vi "Poll Sensor Group 2.vi"(8 "error in":errorcluster, 11 "UART port in":T3) -> (0 "error out":errorcluster, 1 "Timed Out?":bool, 2 "Sensor Group 2":T1={"Infrared"=255, "Buttons"={"Advance"=FALSE, "Play"=FALSE}, "Distance (mm)"=0, "Angle (deg)"=0} {"Infrared" format="%02x"}, 3 "UART port out":T3)   [LabVIEW 2013]
doc: "Poll the iRobot for Sensor Group 2; blocks until response is received, or the operation has timed out.\n\nThis VI both writes to AND reads from the serial port.\n<b>NOTE</b>: This should not be used in a loop if other serial reading or writing VIs are called in parallel loops."
uses:
  Advanced/UART/iRobot UART Port Type.ctl
  Sensor Group 2.ctl
  Buttons.ctl
  Sensor ID.ctl
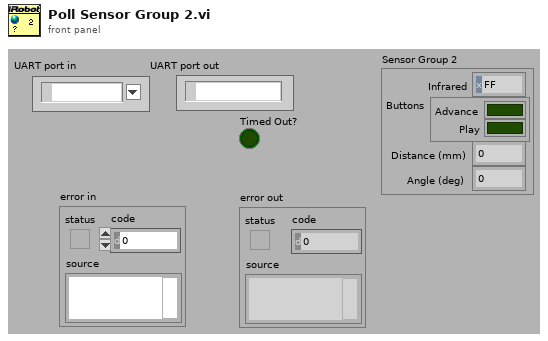
[diagram p1: front panel]
types:
  T1 = typedef "Sensor Group 2.ctl" = cluster{"Infrared":u8, "Buttons":T2, "Distance (mm)":i32, "Angle (deg)":i32}
  T2 = typedef "Buttons.ctl" = cluster{"Advance":bool, "Play":bool}
  T3 = typedef "iRobot UART Port Type.ctl" = refnum<visa-resource-name>
  T4 = typedef "Sensor ID.ctl" = enum8{"Sensor Group 0", "Sensor Group 1", "Sensor Group 2", "Sensor Group 3", "Sensor Group 4", "Sensor Group 5", "Sensor Group 6", "Bump + Wheel Drop", "Wall", "Cliff Left", "Cliff Front Left", "Cliff Front Right", "Cliff Right", "Virtual Wall", "Low Side Driver + Wheel Overcurrent", "Unused 0", "Unused 1", "Infrared", "Buttons", "Distance", "Angle", "Charging State", "Voltage", "Current", "Battery Temperature", "Battery Charge", "Battery Capacity", "Wall Signal", "Cliff Left Signal", "Cliff Front Left Signal", "Cliff Front Right Signal", "Cliff Right Signal", "Cargo Bay Digital Inputs", "Cargo Bay Analog Signal", "Charging Sources Available", "OI Mode", "Song Number", "Song Playing", "Number of Stream Packets", "Requested Velocity", "Requested Radius", "Requested Right Velocity", "Requested Left Velocity"}
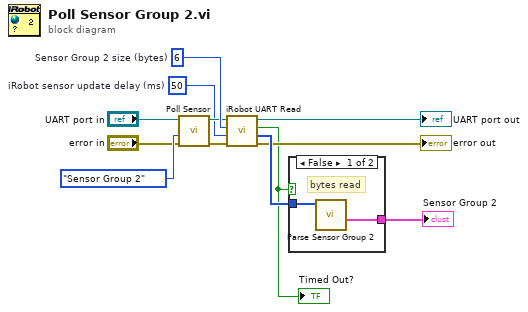
[diagram p0: block diagram]
diagram:
  w3 = 50  # iRobot sensor update delay (ms)
  w11 = 6  # Sensor Group 2 size (bytes)
  n1 = call "Poll Sensor.vi"("error in"="error in", "Sensor ID"=Sensor_ID."Sensor Group 2", "UART port in"="UART port in") -> ("error out"=w6:errorcluster, "UART port out"=w9:T3)  [unwired: 7 in]
  n2 = call "iRobot UART Read.vi"("error in"=w6, "timeout (ms)"=w3, "Number of Bytes"=w11, "UART port in"=w9) -> ("error out"=→"error out":errorcluster, "UART Stream"=w10:u8[], "Timed Out?"=w2:bool, "UART port out"=→"UART port out":T3)  [unwired: 4 in]
  "Timed Out?" <- w2
  n3 = case shown="False" w2 {
    tunnel: w10 -> [w14 _]
    tunnel: [w13 _] -> w1
    frame False {
      # "bytes read"
      n4 = call "Parse Sensor Group 2.vi"("stream in"=w14) -> ("Sensor Group 2"=w13:T1)  [unwired: 9 in, 1 out]
    }
    frame True {
      # "timeout"
    }
  }
  "Sensor Group 2" <- w1
